vi "写入MB session in.vi"(8 "error in (no error)":errorcluster caption="错误输入（无错误）", 10 "MB Serial Master:MB_Master":refnum<class "MB_Master.lvclass">, 11 "HL7输入":refnum<class "HL7.lvclass">) -> (0 "error out":errorcluster caption="错误输出", 3 "HL7输出":refnum<class "HL7.lvclass">)   [LabVIEW 2016, in "HL7.lvlib" / "HL7.lvclass"]
uses:
  HL7.lvclass
  <vilib>/Plasmionique/MB Master/MB_Master/MB_Master.lvclass
  HL7.lvclass/HL7.ctl
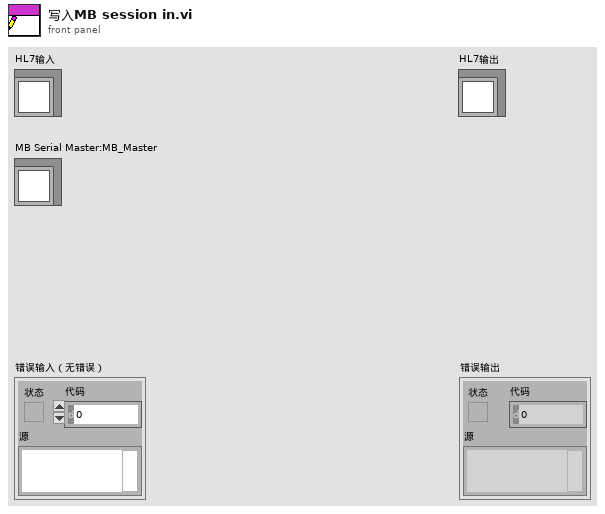
[diagram p1: front panel]
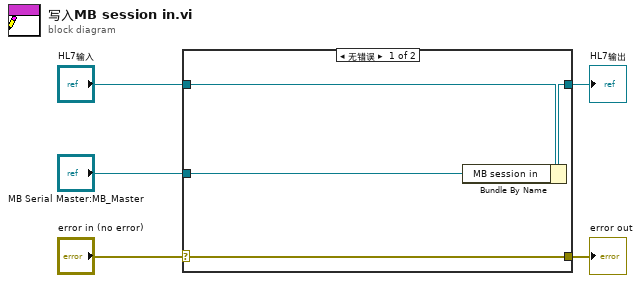
[diagram p0: block diagram]
diagram:
  n1 = case shown="无错误" "error in (no error)" {
    selector: "error in (no error)" -> [w9 w10]
    tunnel: [w9 w10] -> w4
    tunnel: [w7 w11] -> w2
    tunnel: "HL7输入" -> [w8 w11]
    tunnel: "MB Serial Master:MB_Master" -> [w6 _]
    frame No Error {
      n2 = Bundle By Name(cluster=w8, "MB session in"=w6) -> (w7:refnum<class "HL7.lvclass">)
    }
    frame Error {
    }
  }
  "error out" <- w4
  "HL7输出" <- w2
